vi "Control Valve.vi"(0 "Session Handle in":T2, 5 "Valves":T1=17 items=["GV1"=17, "GV2"=18, "GV3"=19, "GV4"=20], 7 "Energize?":bool, 11 "error in (no error)":errorcluster) -> (4 "Session Handle out":T2, 6 "Success?":bool, 8 "Error Code":string, 15 "error out":errorcluster)   [LabVIEW 2015, in "PAS.lvclass"]
uses:
  PAS.lvclass
  Typedefs/Session Handle.ctl
  Typedefs/Valves.ctl
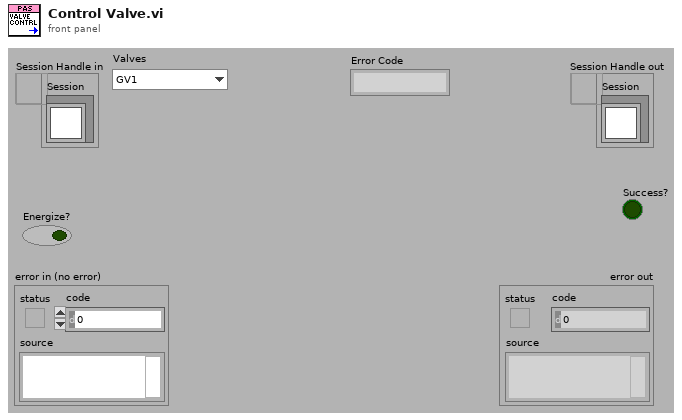
[diagram p1: front panel]
types:
  T1 = typedef "PAS.lvclass/Valves.ctl" = u16
  T2 = typedef "PAS.lvclass/Session Handle.ctl" = refnum<data-value>
  T3 = typedef "XNET Frame CAN.ctl" = cluster{"timestamp":timestamp, "payload":u8[], "identifier":u32, "type":T4, "extended?":bool, "echo?":bool}
  T4 = typedef "XNET Frame Type CAN.ctl" = u8
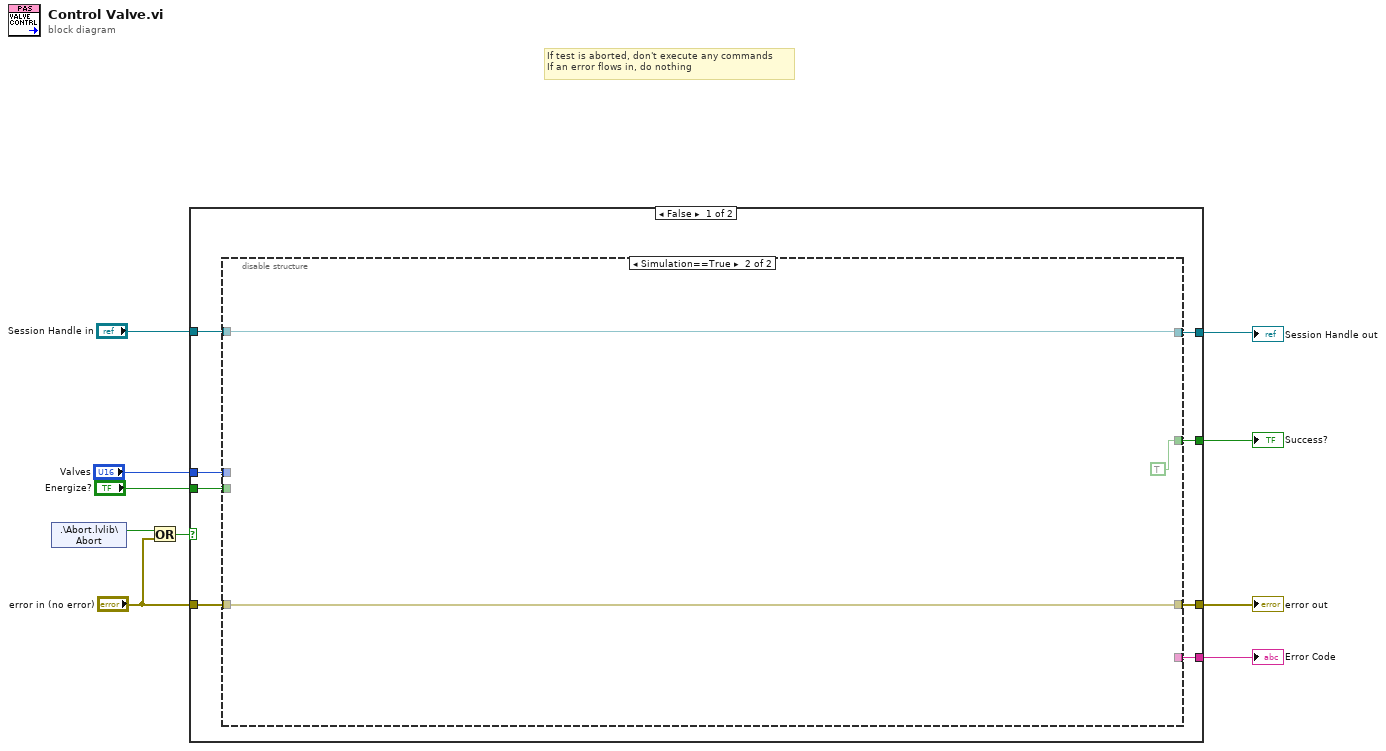
[diagram p0: block diagram]
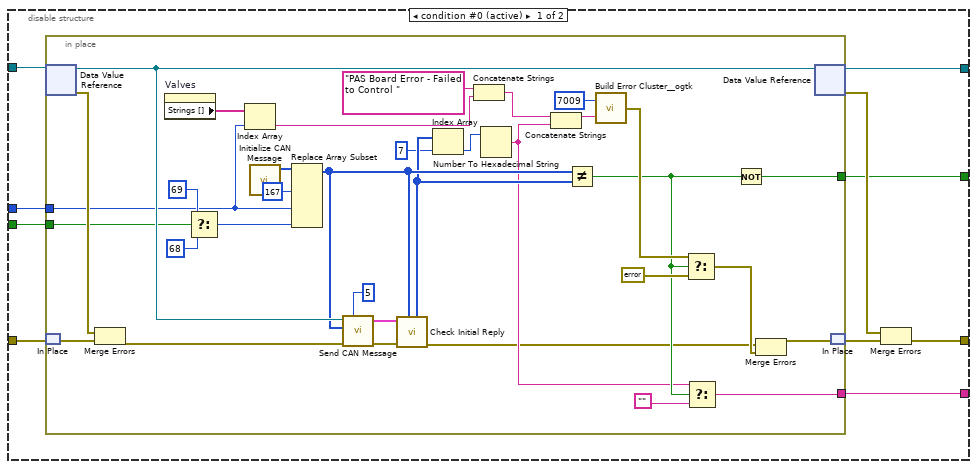
[diagram p2: hidden frame]
diagram:
  # "If test is aborted, don't execute any commands\nIf an error flows in, do nothing"
  n1 = shared-variable ".\\Abort.lvlib\\Abort"() -> (w7:bool)  [unwired: 1 in, 1 out]
  n2 = Or(x=w7, y="error in (no error)") -> (x .or. y?=w5:bool)
  n3 = case shown="False" w5 {
    tunnel: [w18 w67] -> w9
    tunnel: [w17 w66] -> w8
    tunnel: "Session Handle in" -> [w16 w67]
    tunnel: "error in (no error)" -> [w15 w66]
    tunnel: [w14 _] -> w4
    tunnel: "Valves" -> [w13 _]
    tunnel: "Energize?" -> [w12 _]
    tunnel: [w11 _] -> w2
    frame False {
      n4 = disable-structure shown="Simulation==True" {
        disable-tunnel: [w28 w65] -> w18
        disable-tunnel: [w25 w64] -> w17
        disable-tunnel: w16 -> [w24 w65]
        disable-tunnel: w15 -> [w23 w64]
        disable-tunnel: [w22 TRUE] -> w14
        disable-tunnel: w13 -> [w21 _]
        disable-tunnel: w12 -> [w20 _]
        disable-tunnel: [w19 _] -> w11
        frame condition #0 (active) {
          n5 = in-place {
            in-place-border: [w50] -> w22
            in-place-border: w21 -> [w44]
            in-place-border: w20 -> [w49]
            in-place-border: [w32] -> w19
            n6 = in-place-dvr #1(w24) -> (w56:refnum<class "PAS.lvclass">, w59:errorcluster)
            n7 = in-place-match #2(w23) -> (w58:errorcluster)
            n8 = Merge Errors(w59, w58) -> (w57:errorcluster)
            n9 = property on="Valves" class="Ring (strict)"() -> ("Strings []"=w31:string[])  [unwired: 2 in, 2 out]
            n10 = Select(t=u8 69 ("new element/subarray"), s=w49, f=u8 68 ("new element/subarray")) -> (s? t:f=w46:u8)
            n11 = Index Array(array=w31, index=w44) -> (element=w42:string)
            n12 = call "Initialize CAN Message.vi"() -> ("Initial Payload"=w60:u8[])  [unwired: 11 in]
            n13 = Replace Array Subset(array=w60, new element #1=u8 167 ("new element/subarray"), new element #2=w44, new element #3=w46) -> (w45:u8[])  [unwired: 3 in]
            n14 = call "Send CAN Message.vi"("Number of Retries"=5, "error in (no error)"=w57, "payload"=w45, "Gas In"=w56) -> ("error out"=w30:errorcluster, "Reply"=w54:T3[])  [unwired: 5 in, 1 out]
            n15 = call "Check Initial Reply.vi"("Write Message"=w45, "error in (no error)"=w30, "Reply"=w54) -> ("error out"=w29:errorcluster, "Whole Payload"=w40:u8[])  [unwired: 5 in, 2 out]
            n16 = Index Array(array=w40, index=7) -> (element=w38:u8)
            n17 = Concatenate Strings("PAS Board Error - Failed to Control " ("string"), w42) -> (w41:string)
            n18 = Number To Hexadecimal String(2:w38) -> (0:w33:string)  [unwired: 1 in]
            n19 = Concatenate Strings(w41, w33) -> (w37:string)
            n20 = Not Equal?(x=w45, y=w40) -> (x != y?=w34:bool)
            n21 = call <userlib>:"Build Error Cluster__ogtk.vi"("String to Prepend to source (\"\")"=w37, "code"=7009) -> ("error out"=w52:errorcluster)
            n22 = Select(t=w52, s=w34, f=errorcluster {"status"=FALSE, "code"=0, "source"=""}) -> (s? t:f=w36:errorcluster)
            n23 = Select(t=w33, s=w34, f="") -> (s? t:f=w32:string)
            n24 = Not(x=w34) -> (.not. x?=w50:bool)
            n25 = Merge Errors(w29, w36) -> (w61:errorcluster)
            n26 = in-place-dvr #1(w56) -> (w28:T2, w26:errorcluster)
            n27 = in-place-match #2(w61) -> (w27:errorcluster)
          }
          n28 = Merge Errors(w26, w27) -> (w25:errorcluster)
        }
        frame condition #1 {
        }
      }
    }
    frame True {
    }
  }
  "Session Handle out" <- w9
  "error out" <- w8
  "Success?" <- w4
  "Error Code" <- w2
